vi "Generate String.vi"(8 "error in (no error)":errorcluster, 11 "object in":refnum<class "SwitchCaseElement.lvclass">) -> (0 "error out":errorcluster, 2 "String":string, 3 "object out":refnum<class "SwitchCaseElement.lvclass">)   [LabVIEW 2017, in "SwitchCaseElement.lvclass"]
uses:
  SwitchCaseElement.lvclass
  SwitchCaseElement.lvclass/SwitchCaseElement.ctl
  Base/CodeElement.lvclass
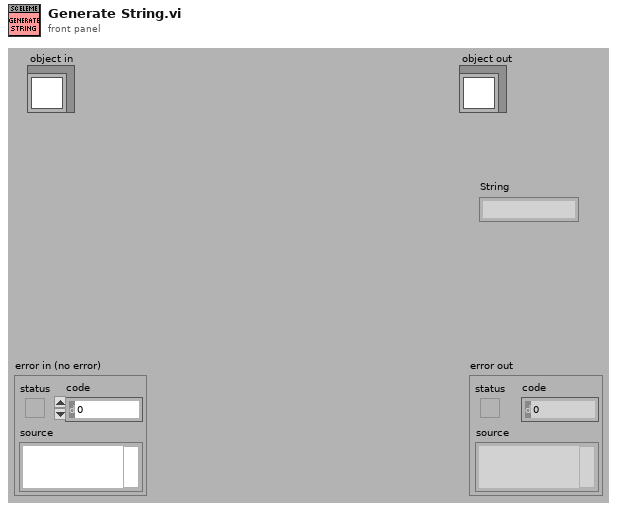
[diagram p1: front panel]
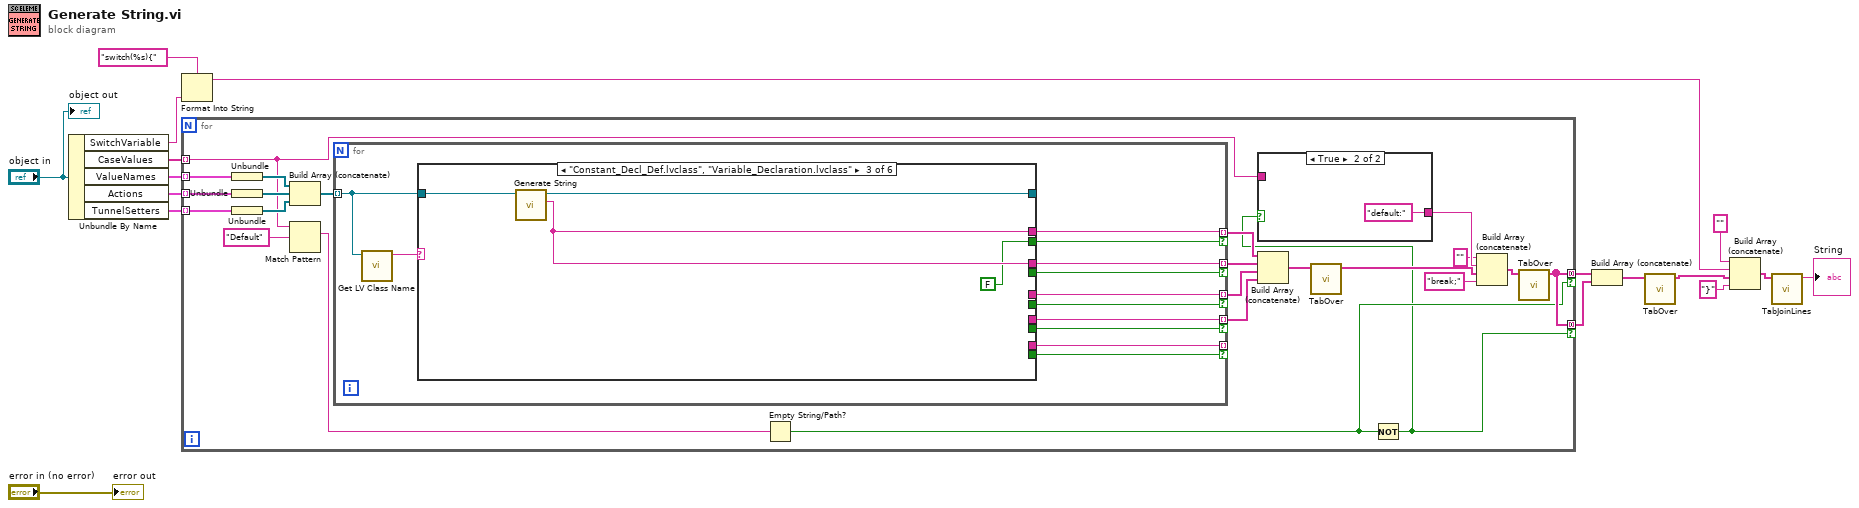
[diagram p0: block diagram]
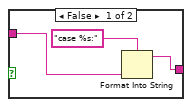
[diagram p2: hidden frame]
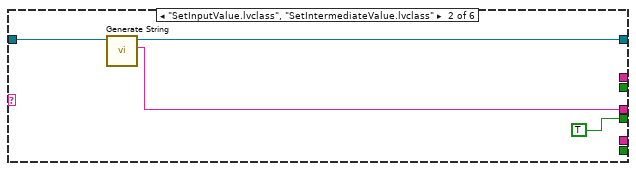
[diagram p4: hidden frame]
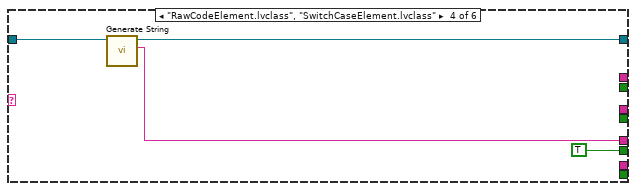
[diagram p5: hidden frame]
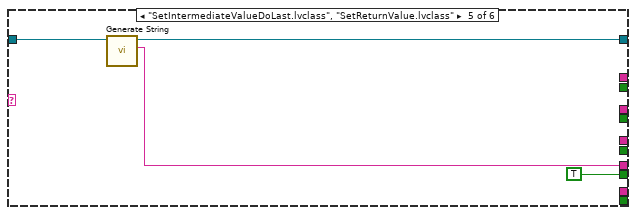
[diagram p6: hidden frame]
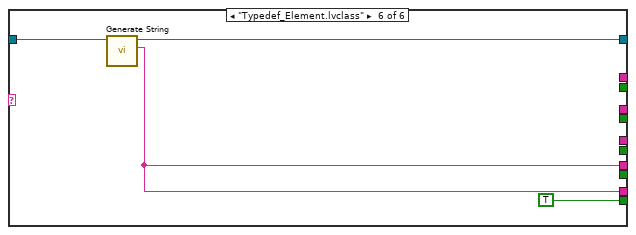
[diagram p7: hidden frame]
diagram:
  n1 = Unbundle By Name("object in") -> ("SwitchVariable"=w14:string, "CaseValues"=w13:string[], "ValueNames"=w12:cluster{refnum<class "CodeElement.lvclass">[]}[], "Actions"=w11:cluster{refnum<class "CodeElement.lvclass">[]}[], "TunnelSetters"=w5:cluster{refnum<class "CodeElement.lvclass">[]}[])
  n2 = Format Into String(format string="switch(%s){", w14) -> (resulting string=w10:string)  [unwired: 2 in, 1 out]
  n3 = for {
    tunnel: w13 -> [w24] mode=indexing
    tunnel: w12 -> [w40] mode=indexing
    tunnel: w11 -> [w39] mode=indexing
    tunnel: [w21] -> w9 mode=concatenating if=w20
    tunnel: w5 -> [w25] mode=indexing
    tunnel: [w21] -> w4 mode=concatenating if=w19
    n4 = Unbundle(w40) -> (w38:refnum<class "CodeElement.lvclass">[])
    n5 = Unbundle(w39) -> (w37:refnum<class "CodeElement.lvclass">[])
    n6 = Unbundle(w25) -> (w26:refnum<class "CodeElement.lvclass">[])
    n7 = Build Array (concatenate)(w38, w37, w26) -> (w36:refnum<class "CodeElement.lvclass">[])
    n8 = Match Pattern(string=w24, regular expression="Default") -> (match substring=w22:string)  [unwired: 1 in, 3 out]
    n9 = for {
      tunnel: w36 -> [w55] mode=indexing
      tunnel: [w54] -> w35 mode=indexing if=w53
      tunnel: [w52] -> w34 mode=indexing if=w51
      tunnel: [w50] -> w33 mode=indexing if=w49
      tunnel: [w48] -> _ mode=indexing if=w47
      tunnel: [w46] -> w32 mode=indexing if=w45
      n10 = call <vilib>:"Get LV Class Name.vi"("object"=w55) -> ("class name"=w56:string)  [unwired: 9 in, 1 out]
      n11 = case shown="\"Constant_Decl_Def.lvclass\", \"Variable_Declaration.lvclass\"" w56 {
        tunnel: [w57 w60 w64 w68 w72 w76] -> _
        tunnel: w55 -> [w57 w61 w65 w69 w73 w77]
        tunnel: [_ w59 w63 _ _ _] -> w54
        tunnel: [_ TRUE _ _ _ _] -> w53
        tunnel: [_ _ _ w67 _ _] -> w52
        tunnel: [_ _ _ TRUE _ _] -> w51
        tunnel: [_ _ _ _ TRUE _] -> w49
        tunnel: [_ _ _ _ w70 w75] -> w50
        tunnel: [_ _ _ _ _ w75] -> w48
        tunnel: [_ _ _ _ _ TRUE] -> w47
        tunnel: [_ _ w63 _ _ _] -> w46
        tunnel: [_ _ FALSE _ _ _] -> w45
        frame "False", Default {
        }
        frame "SetInputValue.lvclass", "SetIntermediateValue.lvclass" {
          n12 = call-dynamic "Generate String.vi"("object in"=w61) -> ("String"=w59:string, "object out"=w60:refnum<class "CodeElement.lvclass">)  [unwired: 8 in, 1 out]
        }
        frame "Constant_Decl_Def.lvclass", "Variable_Declaration.lvclass" {
          n13 = call-dynamic "Generate String.vi"("object in"=w65) -> ("String"=w63:string, "object out"=w64:refnum<class "CodeElement.lvclass">)  [unwired: 8 in, 1 out]
        }
        frame "RawCodeElement.lvclass", "SwitchCaseElement.lvclass" {
          n14 = call-dynamic "Generate String.vi"("object in"=w69) -> ("String"=w67:string, "object out"=w68:refnum<class "CodeElement.lvclass">)  [unwired: 8 in, 1 out]
        }
        frame "SetIntermediateValueDoLast.lvclass", "SetReturnValue.lvclass" {
          n15 = call-dynamic "Generate String.vi"("object in"=w73) -> ("String"=w70:string, "object out"=w72:refnum<class "CodeElement.lvclass">)  [unwired: 8 in, 1 out]
        }
        frame "Typedef_Element.lvclass" {
          n16 = call-dynamic "Generate String.vi"("object in"=w77) -> ("String"=w75:string, "object out"=w76:refnum<class "CodeElement.lvclass">)  [unwired: 8 in, 1 out]
        }
      }
    }
    n17 = Empty String/Path?(string/path=w22) -> (empty?=w20:bool)
    n18 = Build Array (concatenate)(w32, w35, w34, w33) -> (w31:string[])
    n19 = call "TabOver.vi"("Array in"=w31) -> ("Array out"=w30:string[])  [unwired: 10 in]
    n20 = Not(x=w20) -> (.not. x?=w19:bool)
    n21 = case shown="True" w19 {
      tunnel: [w42 "default:"] -> w29
      tunnel: w24 -> [w41 _]
      frame False {
        n22 = Format Into String(format string="case %s:", w41) -> (resulting string=w42:string)  [unwired: 2 in, 1 out]
      }
      frame True {
      }
    }
    n23 = Build Array (concatenate)("" ("element"), w29, w30, "break;" ("format string")) -> (w27:string[])
    n24 = call "TabOver.vi"("Array in"=w27) -> ("Array out"=w21:string[])  [unwired: 10 in]
  }
  n25 = Build Array (concatenate)(w9, w4) -> (w3:string[])
  n26 = call "TabOver.vi"("Array in"=w3) -> ("Array out"=w2:string[])  [unwired: 10 in]
  n27 = Build Array (concatenate)("" ("element"), w10, w2, "}" ("format string")) -> (w7:string[])
  n28 = call "TabJoinLines.vi"("Array"=w7) -> ("String"=→"String":string)  [unwired: 10 in]
  "error out" <- "error in (no error)"
  "object out" <- "object in"
